vi "Insert Item.vi"(8 "error in (no error)":errorcluster, 9 "After item":string, 10 "Item":string, 11 "Interactive Tree in":refnum<class "Sequence Controller.lvclass">) -> (0 "error out":errorcluster, 3 "Interactive Tree out":refnum<class "Sequence Controller.lvclass">)   [LabVIEW 2016, in "Sequence Controller.lvclass"]
uses:
  Sequence Controller.lvclass
  Sequence Controller.lvclass/Sequence Controller.ctl
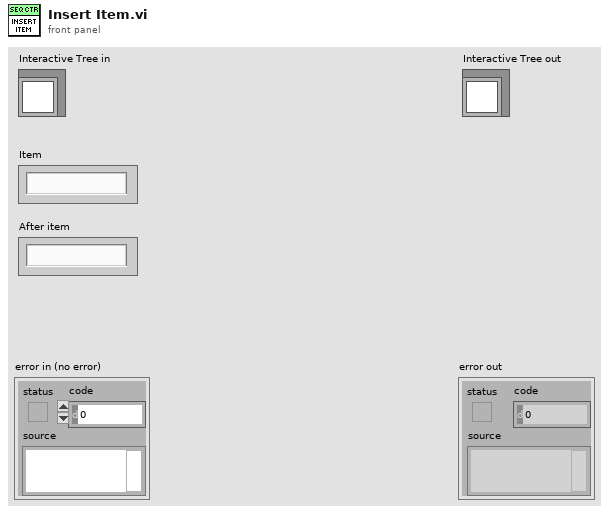
[diagram p1: front panel]
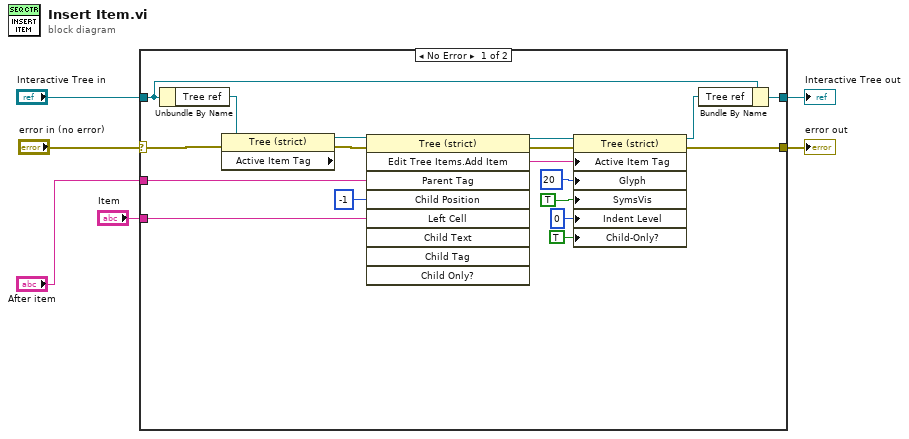
[diagram p0: block diagram]
diagram:
  n1 = case shown="No Error" "error in (no error)" {
    selector: "error in (no error)" -> [w20 w26]
    tunnel: [w11 w26] -> w5
    tunnel: [w19 w25] -> w3
    tunnel: "Interactive Tree in" -> [w24 w25]
    tunnel: "Item" -> [w17 _]
    tunnel: "After item" -> [w9 _]
    frame No Error {
      n2 = Unbundle By Name(w24) -> ("Tree ref"=w23:refnum<vi>)
      n3 = property class="Tree (strict)" props=["Active Item Tag"](reference=w23, error in=w20) -> (reference out=w10:refnum<vi>, error out=w22:errorcluster)  [unwired: 1 out]
      n4 = invoke class="Tree (strict)" method="Edit Tree Items.Add Item"(reference=w10, error in=w22, "Parent Tag"=w9, "Child Position"=-1, "Left Cell"=w17) -> (reference out=w18:refnum<vi>, error out=w12:errorcluster, "Edit Tree Items:Add Item"=w15:string)  [unwired: 4 in, 6 out]
      n5 = property class="Tree (strict)"(reference=w18, error in=w12, "Active Item Tag"=w15, "Glyph"=20 ("Active Item:Symbol Index"), "SymsVis"=TRUE ("Visible Items:Symbols Visible"), "Indent Level"=0 ("Active Item:Indent Level"), "Child-Only?"=TRUE ("Active Item:Child-Only?")) -> (reference out=w16:refnum<vi>, error out=w11:errorcluster)
      n6 = Bundle By Name(cluster=w24, "Tree ref"=w16) -> (w19:refnum<class "Sequence Controller.lvclass">)
    }
    frame Error {
    }
  }
  "error out" <- w5
  "Interactive Tree out" <- w3
